vi "Teleop.vi"(10 "Match Info":T1={"Autonomous Elapsed Seconds"=0.0, "TeleOp Elapsed Seconds"=0.0, "Disabled Elapsed Seconds"=0.0, "Visited Autonomous"=FALSE, "Visited TeleOp"=FALSE, "Visited Disabled"=FALSE, "Autonomous Settings"={"Autonomous Style"=enum."Independent", "VI Refnum"=refnum}}, 11 "Call Context":T2) -> ()   [LabVIEW 2012]
doc: "This VI is called for each TeleOp packet received from the DS where the robot is not disabled. It is often used to read from the joysticks and update I/O or to update setpoints for timed control loops. It should complete and return within 20 milliseconds or it may miss DS packets."
uses:
  <vilib>/Rock Robotics/WPI/DriverStation/WPI_DriverStationDerivedRobotMode.ctl
  <vilib>/Rock Robotics/WPI/DriverStation/WPI_DriverStationMatch Info.ctl
  Robot Global Data.vi
  <vilib>/Rock Robotics/WPI/Joystick/WPI_JoystickGetSetRefNum.vi
  <vilib>/Rock Robotics/WPI/RobotDrive/WPI_RobotDriveGetSetRefNum.vi
  <vilib>/Rock Robotics/WPI/Solenoid/WPI_SolenoidSetEnum.vi
  <vilib>/Rock Robotics/WPI/Solenoid/WPI_SolenoidValue.ctl
panel:
  out "Numeric 1":dbl(slide) scale=0.0..100.0
  out "Boolean 2":bool
  out "Boolean 1":bool
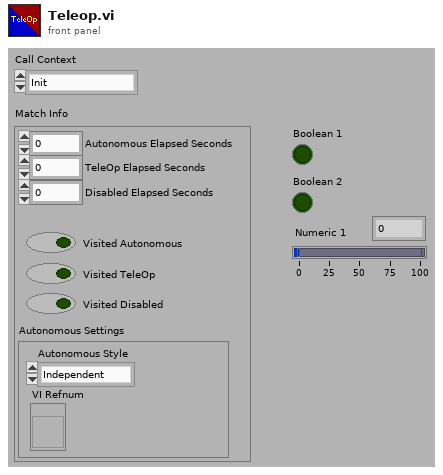
[diagram p1: front panel]
types:
  T1 = typedef "WPI_DriverStationMatch Info.ctl" = cluster{"Autonomous Elapsed Seconds":dbl, "TeleOp Elapsed Seconds":dbl, "Disabled Elapsed Seconds":dbl, "Visited Autonomous":bool, "Visited TeleOp":bool, "Visited Disabled":bool, "Autonomous Settings":cluster{"Autonomous Style":enum16{"Iterative", "Independent"}, "VI Refnum":refnum<vi>}}
  T2 = typedef "WPI_DriverStationDerivedRobotMode.ctl" = enum16{"Init", "Execute", "Stop"}
  T3 = typedef "WPI_JoystickDevRef.ctl" = cluster{"Device":T4}
  T4 = typedef "WPI_JoystickDeviceEnum.ctl" = enum16{"USB 1", "USB 2", "USB 3", "USB 4", "Kinect 1", "Kinect 2"}
  T5 = typedef "WPI_JoystickButtonState.ctl" = cluster{"Button 1":bool, "Button 2":bool, "Button 3":bool, "Button 4":bool, "Button 5":bool, "Button 6":bool, "Button 7":bool, "Button 8":bool, "Button 9":bool, "Button 10":bool, "Button 11":bool, "Button 12":bool}
  T6 = cluster{"axis 1 (x)":dbl, "axis 2 (y)":dbl, "axis 3 (throttle)":dbl, "axis 4":dbl, "axis 5":dbl, "axis 6":dbl}
  T7 = typedef "WPI_RobotDriveDevRef.ctl" = cluster{"DevStatus":errorcluster, "Motors[]":T8[], "Square Inputs":bool, "Max Output":dbl, "Isochronous":bool}
  T8 = typedef "WPI_MotorControlDeviceRef.ctl" = cluster{"DeviceStatus":errorcluster, "Type":enum16{"PWM", "CAN"}, "PWM":cluster{"Digital Module":T9, "PWM Channel":T10, "DeadBand":T11}, "CAN":cluster{"Device Number":u8, "Control Mode":T12, "Semaphore":T13, "Max Vout":dbl}, "Invert":bool, "TransformRef":T14, "InvTransformRef":T14}
  T9 = typedef "FPGA_TypedefDigitalModule.ctl" = enum16{"Digital Module 1", "Digital Module 2"}
  T10 = typedef "FPGA_DIOPWMChannel.ctl" = enum8{"PWM 1", "PWM 2", "PWM 3", "PWM 4", "PWM 5", "PWM 6", "PWM 7", "PWM 8", "PWM 9", "PWM 10", "Invalid"}
  T11 = typedef "WPI_PWMDeadband.ctl" = cluster{"Name":string, "maxPositivePwm":i32, "minPositivePwm":i32, "centerPwm":i32, "maxNegativePwm":i32, "minNegativePwm":i32, "angularRange":u16}
  T12 = typedef "WPI_CANJaguar_ControlMode.ctl" = enum8{"Percent VBus", "Current", "Speed", "Position", "Voltage"}
  T13 = typedef "Semaphore RefNum" = refnum<k1>
  T14 = typedef "WPI_PWMTransform_ConPane.ctl" = refnum<vi>
  T15 = typedef "WPI_SolenoidValue.ctl" = enum16{"Off", "On", "Forward", "Reverse"}
  T16 = typedef "WPI_SolenoidDevRef.ctl" = cluster{"DevStatus":errorcluster, "Solenoid Module":T17, "Forward Solenoid Channel":T18, "Reverse Solenoid Channel":T18}
  T17 = typedef "FPGA_TypedefSolenoidModule.ctl" = enum16{"Solenoid Module 1", "Solenoid Module 2"}
  T18 = typedef "WPI_SolenoidChannel.ctl" = enum8{"Solenoid 1", "Solenoid 2", "Solenoid 3", "Solenoid 4", "Solenoid 5", "Solenoid 6", "Solenoid 7", "Solenoid 8", "Invalid"}
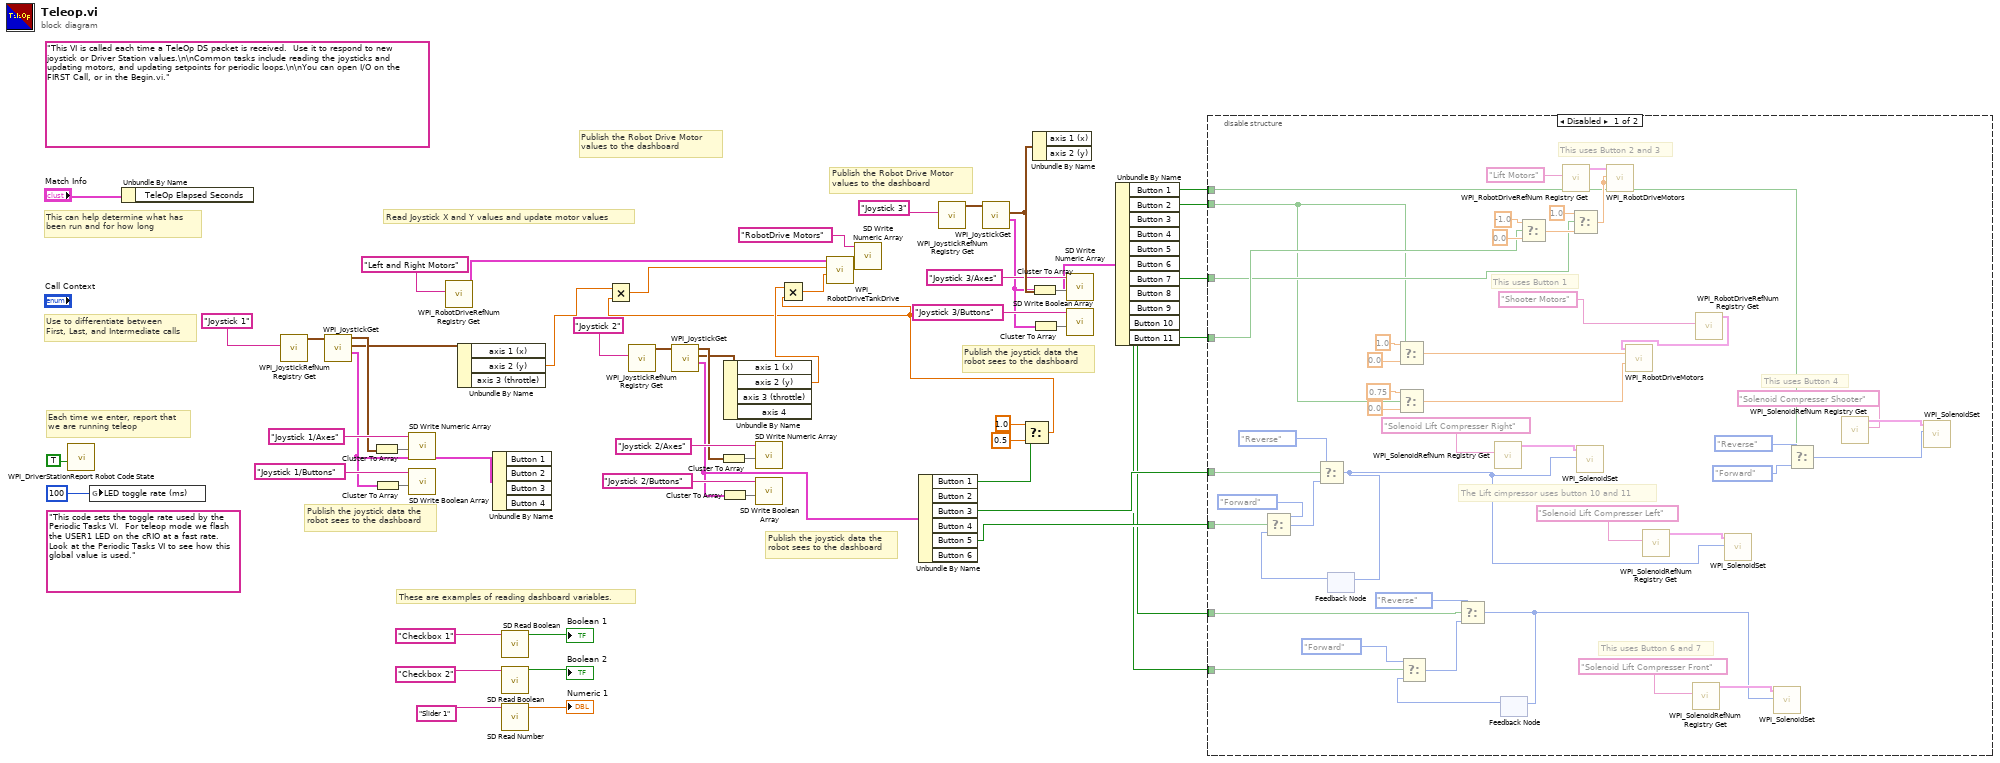
[diagram p0: block diagram]
diagram:
  (unwired) "This code sets the toggle rate used by the Periodic Tasks VI.  For teleop mode we flash the USER1 LED on the cRIO at a fast rate.  Look at the Periodic Tasks VI to see how this global value is used."
  (unwired) "This VI is called each time a TeleOp DS packet is received.  Use it to respond to new joystick or Driver Station values.\n\nCommon tasks include reading the joysticks and updating motors, and updating setpoints for periodic loops.\n\nYou can open I/O on the FIRST Call, or in the Begin.vi."
  # "Publish the joystick data the\nrobot sees to the dashboard"
  # "Publish the Robot Drive Motor\nvalues to the dashboard"
  # "Publish the joystick data the\nrobot sees to the dashboard"
  # "These are examples of reading dashboard variables."
  # "Publish the Robot Drive Motor\nvalues to the dashboard"
  # "Publish the joystick data the\nrobot sees to the dashboard"
  # "Each time we enter, report that\nwe are running teleop"
  # "Use to differentiate between\nFirst, Last, and Intermediate calls"
  # "This can help determine what has\nbeen run and for how long"
  # "Read Joystick X and Y values and update motor values"
  n1 = call <vilib>:"WPI_DriverStationReport Robot Code State.vi"("TeleOp"=TRUE ("Autonomous")) -> ()  [unwired: 10 in, 1 out]
  n2 = global write "Robot Global Data.vi" "LED toggle rate (ms)"(u32 100 ("LED ms toggle rate")) -> ()
  n3 = Unbundle By Name("Match Info") -> ()  [unwired: 1 out]
  n4 = call <vilib>:"WPI_JoystickRefNum Registry Get.vi"("refnum name"="Joystick 1") -> ("JoystickDevRef"=w51:T3)  [unwired: 1 in, 9 out]
  n5 = call <vilib>:"WPI_JoystickGet.vi"("JoystickDevRef"=w51) -> ("Buttons"=w20:T5, "Axes"=w17:T6, "JoystickDevRef"=w22:T3)  [unwired: 1 in, 3 out]
  n6 = Cluster To Array(cluster=w22) -> (array=w46:T4[])
  n7 = Cluster To Array(cluster=w20) -> (array=w48:bool[])
  n8 = call <vilib>:"SD Write Numeric Array.vi"("Numeric Array"=w46, "Name"="Joystick 1/Axes") -> ()  [unwired: 8 in, 2 out]
  n9 = call <vilib>:"SD Write Boolean Array.vi"("Boolean Array"=w48, "Name"="Joystick 1/Buttons") -> ()  [unwired: 8 in, 2 out]
  n10 = call <vilib>:"WPI_RobotDriveRefNum Registry Get.vi"("refnum name"="Left and Right Motors") -> ("RobotDriveDevRef"=w53:T7)  [unwired: 1 in, 9 out]
  n11 = Unbundle By Name(w17) -> ("axis 2 (y)"=w3:dbl)  [unwired: 2 out]
  n12 = Unbundle By Name(w20) -> ()  [unwired: 4 out]
  n13 = call <vilib>:"SD Read Boolean.vi"("Name"="Checkbox 1" ("refnum name")) -> ("Boolean"=→"Boolean 1":bool)  [unwired: 8 in, 2 out]
  n14 = call <vilib>:"SD Read Boolean.vi"("Name"="Checkbox 2" ("refnum name")) -> ("Boolean"=→"Boolean 2":bool)  [unwired: 8 in, 2 out]
  n15 = call <vilib>:"SD Read Number.vi"("Name"="Slider 1" ("refnum name")) -> ("Numeric"=→"Numeric 1":dbl)  [unwired: 8 in, 2 out]
  n16 = call <vilib>:"WPI_JoystickRefNum Registry Get.vi"("refnum name"="Joystick 2") -> ("JoystickDevRef"=w33:T3)  [unwired: 1 in, 9 out]
  n17 = call <vilib>:"WPI_JoystickGet.vi"("JoystickDevRef"=w33) -> ("Buttons"=w19:T5, "Axes"=w18:T6, "JoystickDevRef"=w21:T3)  [unwired: 1 in, 3 out]
  n18 = Cluster To Array(cluster=w21) -> (array=w23:T4[])
  n19 = Cluster To Array(cluster=w19) -> (array=w34:bool[])
  n20 = Unbundle By Name(w18) -> ("axis 2 (y)"=w5:dbl)  [unwired: 3 out]
  n21 = call <vilib>:"SD Write Numeric Array.vi"("Numeric Array"=w23, "Name"="Joystick 2/Axes") -> ()  [unwired: 8 in, 2 out]
  n22 = call <vilib>:"SD Write Boolean Array.vi"("Boolean Array"=w34, "Name"="Joystick 2/Buttons") -> ()  [unwired: 8 in, 2 out]
  n23 = Unbundle By Name(w19) -> ("Button 1"=w8:bool, "Button 3"=w15:bool, "Button 5"=w16:bool)  [unwired: 3 out]
  n24 = call <vilib>:"WPI_JoystickRefNum Registry Get.vi"("refnum name"="Joystick 3") -> ("JoystickDevRef"=w30:T3)  [unwired: 1 in, 9 out]
  n25 = call <vilib>:"WPI_JoystickGet.vi"("JoystickDevRef"=w30) -> ("Buttons"=w24:T5, "Axes"=w27:T6)  [unwired: 1 in, 4 out]
  n26 = Select(t=1.0, s=w8, f=0.5) -> (s? t:f=w2:dbl)
  n27 = Multiply(x=w3, y=w2) -> (x*y=w1:dbl)
  n28 = Multiply(x=w5, y=w2) -> (x*y=w4:dbl)
  n29 = call <vilib>:"WPI_RobotDriveTankDrive.vi"("Right axis value"=w4, "Left axis value"=w1, "RobotDriveDevRef"=w53) -> ("Motor Values"=w43:dbl[])  [unwired: 6 in, 2 out]
  n30 = call <vilib>:"SD Write Numeric Array.vi"("Numeric Array"=w43, "Name"="RobotDrive Motors") -> ()  [unwired: 8 in, 2 out]
  n31 = Cluster To Array(cluster=w27) -> (array=w26:dbl[])
  n32 = Cluster To Array(cluster=w24) -> (array=w29:bool[])
  n33 = Unbundle By Name(w27) -> ()  [unwired: 2 out]
  n34 = call <vilib>:"SD Write Numeric Array.vi"("Numeric Array"=w26, "Name"="Joystick 3/Axes") -> ()  [unwired: 8 in, 2 out]
  n35 = call <vilib>:"SD Write Boolean Array.vi"("Boolean Array"=w29, "Name"="Joystick 3/Buttons") -> ()  [unwired: 8 in, 2 out]
  n36 = Unbundle By Name(w24) -> ("Button 1"=w11:bool, "Button 2"=w12:bool, "Button 4"=w9:bool, "Button 6"=w10:bool, "Button 7"=w13:bool, "Button 11"=w14:bool)  [unwired: 5 out]
  n37 = disable-structure shown="Disabled" {
    disable-tunnel: w16 -> [w63 _]
    disable-tunnel: w15 -> [w62 _]
    disable-tunnel: w14 -> [w61 _]
    disable-tunnel: w13 -> [w60 _]
    disable-tunnel: w12 -> [w59 _]
    disable-tunnel: w11 -> [w58 _]
    disable-tunnel: w10 -> [w57 _]
    disable-tunnel: w9 -> [w56 _]
    frame Disabled {
      # "This uses Button 2 and 3"
      # "The Lift cimpressor uses button 10 and 11"
      # "This uses Button 1"
      # "This uses Button 6 and 7"
      # "This uses Button 4"
      n38 = feedback #1() -> (w73:T15)  [unwired: 1 in]
      n39 = Select(t=WPI_SolenoidValue."Forward" ("Value"), s=w63, f=w73) -> (s? t:f=w72:T15)
      n40 = Select(t=WPI_SolenoidValue."Reverse" ("Value"), s=w62, f=w72) -> (s? t:f=w69:T15)
      n41 = feedback-in #1(w69) -> ()
      n42 = Select(t=1.0, s=w59, f=0.0) -> (s? t:f=w94:dbl)
      n43 = Select(t=0.75 ("t 2"), s=w59, f=0.0) -> (s? t:f=w95:dbl)
      n44 = call <vilib>:"WPI_SolenoidRefNum Registry Get.vi"("refnum name"="Solenoid Lift Compresser Right") -> ("SolenoidDevRef"=w83:T16)  [unwired: 9 in, 1 out]
      n45 = feedback #2() -> (w74:T15)  [unwired: 1 in]
      n46 = Select(t=WPI_SolenoidValue."Forward" ("Value"), s=w57, f=w74) -> (s? t:f=w76:T15)
      n47 = Select(t=WPI_SolenoidValue."Reverse" ("Value"), s=w56, f=w76) -> (s? t:f=w75:T15)
      n48 = feedback-in #2(w75) -> ()
      n49 = Select(t=-1.0, s=w61, f=0.0) -> (s? t:f=w88:dbl)
      n50 = call <vilib>:"WPI_RobotDriveRefNum Registry Get.vi"("refnum name"="Lift Motors") -> ("RobotDriveDevRef"=w86:T7)  [unwired: 9 in, 1 out]
      n51 = Select(t=1.0, s=w60, f=w88) -> (s? t:f=w85:dbl)
      n52 = call-poly <vilib>:"WPI_SolenoidSet.vi"("Value"=w69, "SolenoidDevRef"=w83) -> ()  [unwired: 8 in, 2 out]
      n53 = call <vilib>:"WPI_RobotDriveMotors.vi"("RightSpeed"=w85, "LeftSpeed"=w85, "RobotDriveDevRef"=w86) -> ()  [unwired: 1 in, 8 out]
      n54 = call <vilib>:"WPI_SolenoidRefNum Registry Get.vi"("refnum name"="Solenoid Lift Compresser Left") -> ("SolenoidDevRef"=w82:T16)  [unwired: 9 in, 1 out]
      n55 = call <vilib>:"WPI_SolenoidRefNum Registry Get.vi"("refnum name"="Solenoid Lift Compresser Front") -> ("SolenoidDevRef"=w78:T16)  [unwired: 9 in, 1 out]
      n56 = call <vilib>:"WPI_RobotDriveRefNum Registry Get.vi"("refnum name"="Shooter Motors") -> ("RobotDriveDevRef"=w92:T7)  [unwired: 9 in, 1 out]
      n57 = call <vilib>:"WPI_RobotDriveMotors.vi"("RightSpeed"=w95, "LeftSpeed"=w94, "RobotDriveDevRef"=w92) -> ()  [unwired: 1 in, 8 out]
      n58 = call-poly <vilib>:"WPI_SolenoidSet.vi"("Value"=w69, "SolenoidDevRef"=w82) -> ()  [unwired: 8 in, 2 out]
      n59 = call-poly <vilib>:"WPI_SolenoidSet.vi"("Value"=w75, "SolenoidDevRef"=w78) -> ()  [unwired: 8 in, 2 out]
      n60 = Select(t=WPI_SolenoidValue."Reverse" ("Value"), s=w58, f=WPI_SolenoidValue."Forward" ("Value")) -> (s? t:f=w64:T15)
      n61 = call <vilib>:"WPI_SolenoidRefNum Registry Get.vi"("refnum name"="Solenoid Compresser Shooter") -> ("SolenoidDevRef"=w68:T16)  [unwired: 9 in, 1 out]
      n62 = call-poly <vilib>:"WPI_SolenoidSet.vi"("Value"=w64, "SolenoidDevRef"=w68) -> ()  [unwired: 8 in, 2 out]
    }
    frame Enabled {
    }
  }
